vi "myDAQ Progression.vi"() -> ()   [LabVIEW 2010]
doc: "NI-K12 Lab style progress page with 5 parts."
uses:
  ActivityGuideEvents.ctl
  Utilities/myDAQ_State.ctl
  Utilities/AG Tab Action.ctl
  Utilities/myDAQmx/myDAQmx Create Channel/Create myDAQ AI.vi
  Utilities/myDAQmx/myDAQmx Read/myDAQmx Read Analog Value.vi
panel:
  in  "Reconnect to myDAQ":bool
  out "Connected":bool
  out "Searching for myDAQ":bool
  in  "Progress Bar":T1(radio)=enum."Apply 4"
  in  "Focus":bool
  in  "stop":bool
  in  "Leave":bool
  in  "Resources":path[](array[path])
  in  "TabButtonsRef":refnum<vi>
  out "DAQ error Info":string
  out "Error Count":u32
  out "Error Out":errorcluster
  out "Current State":T2=enum."Disconnect"
  out "DAQ Loop":i32=548
  in  "ActivityGuideEvents":T3
  in  "Tab Control":T4(tab)=enum."Part 3"
  out "Value 0":dbl
  out "Part 5":dbl
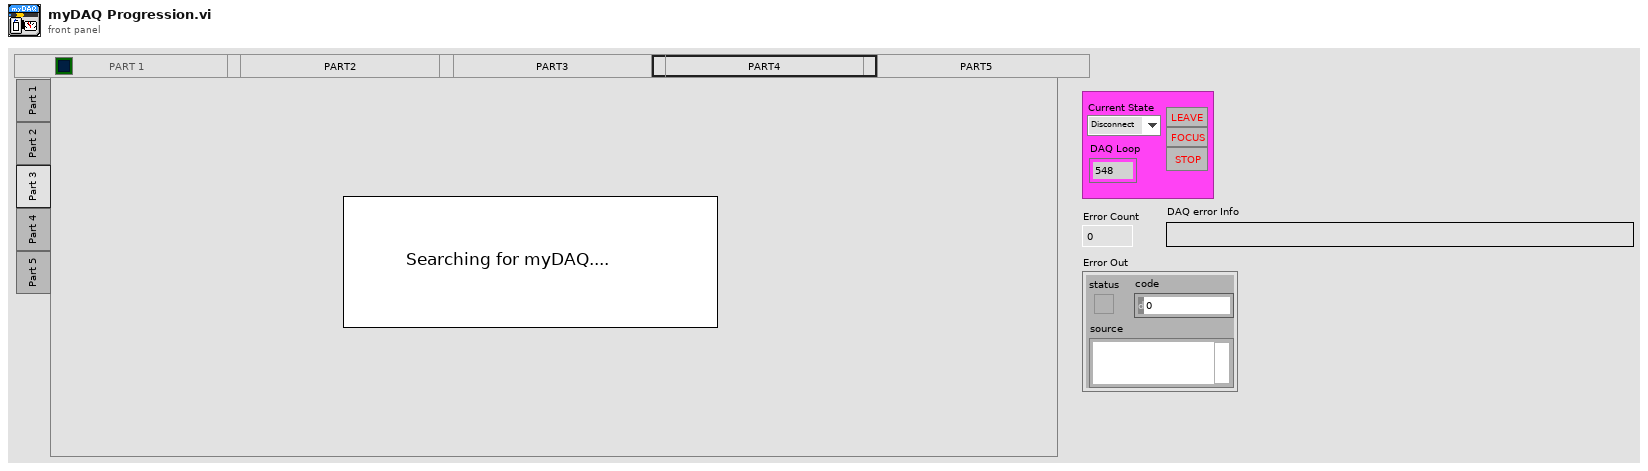
[diagram p1: front panel]
types:
  T1 = enum32{"Apply", "Apply 2", "Apply 3", "Apply 4", "Apply 5"}
  T2 = typedef "myDAQ_State.ctl" = enum16{"Initilize", "Connect", "Calibrate", "Communicate", "Wait", "Disconnect", "Error", "Close"}
  T3 = typedef "ActivityGuideEvents.ctl" = refnum<event-registration>
  T4 = enum32{"Part 1", "Part 2", "Part 3", "Part 4", "Part 5"}
  T5 = typedef "AG Tab Action.ctl" = enum16{"Initilize", "Select", "Blink", "Disable", "KeyFocus", "Set Description", "Hide", "NULL"}
  T6 = typedef "eventvkey.ctl" = enum16{"ASCII", "Enter", "Return", "Shift", "Ctrl", "Alt", "Cmd", "Opt", "Caps", "NumLock", "Clear", "Break", "Up", "Down", "Left", "Right", "Insert", "Delete", "Home", "End", "PageUp", "PageDown", "Escape", "Help", "Pause", "ScrollLock", "F1", "F2", "F3", "F4", "F5", "F6", "F7", "F8", "F9", "F10", "F11", "F12", "F13", "F14", "F15", "F16", "F17", "F18", "F19", "F20", "F21", "F22", "F23", "F24", "Play", "VolumeUp", "VolumeDown", "Mute", "Two Byte Char"}
  T7 = cluster{"Shift":bool, "Ctrl":bool, "Alt":bool, "Cmd":bool, "Opt":bool}
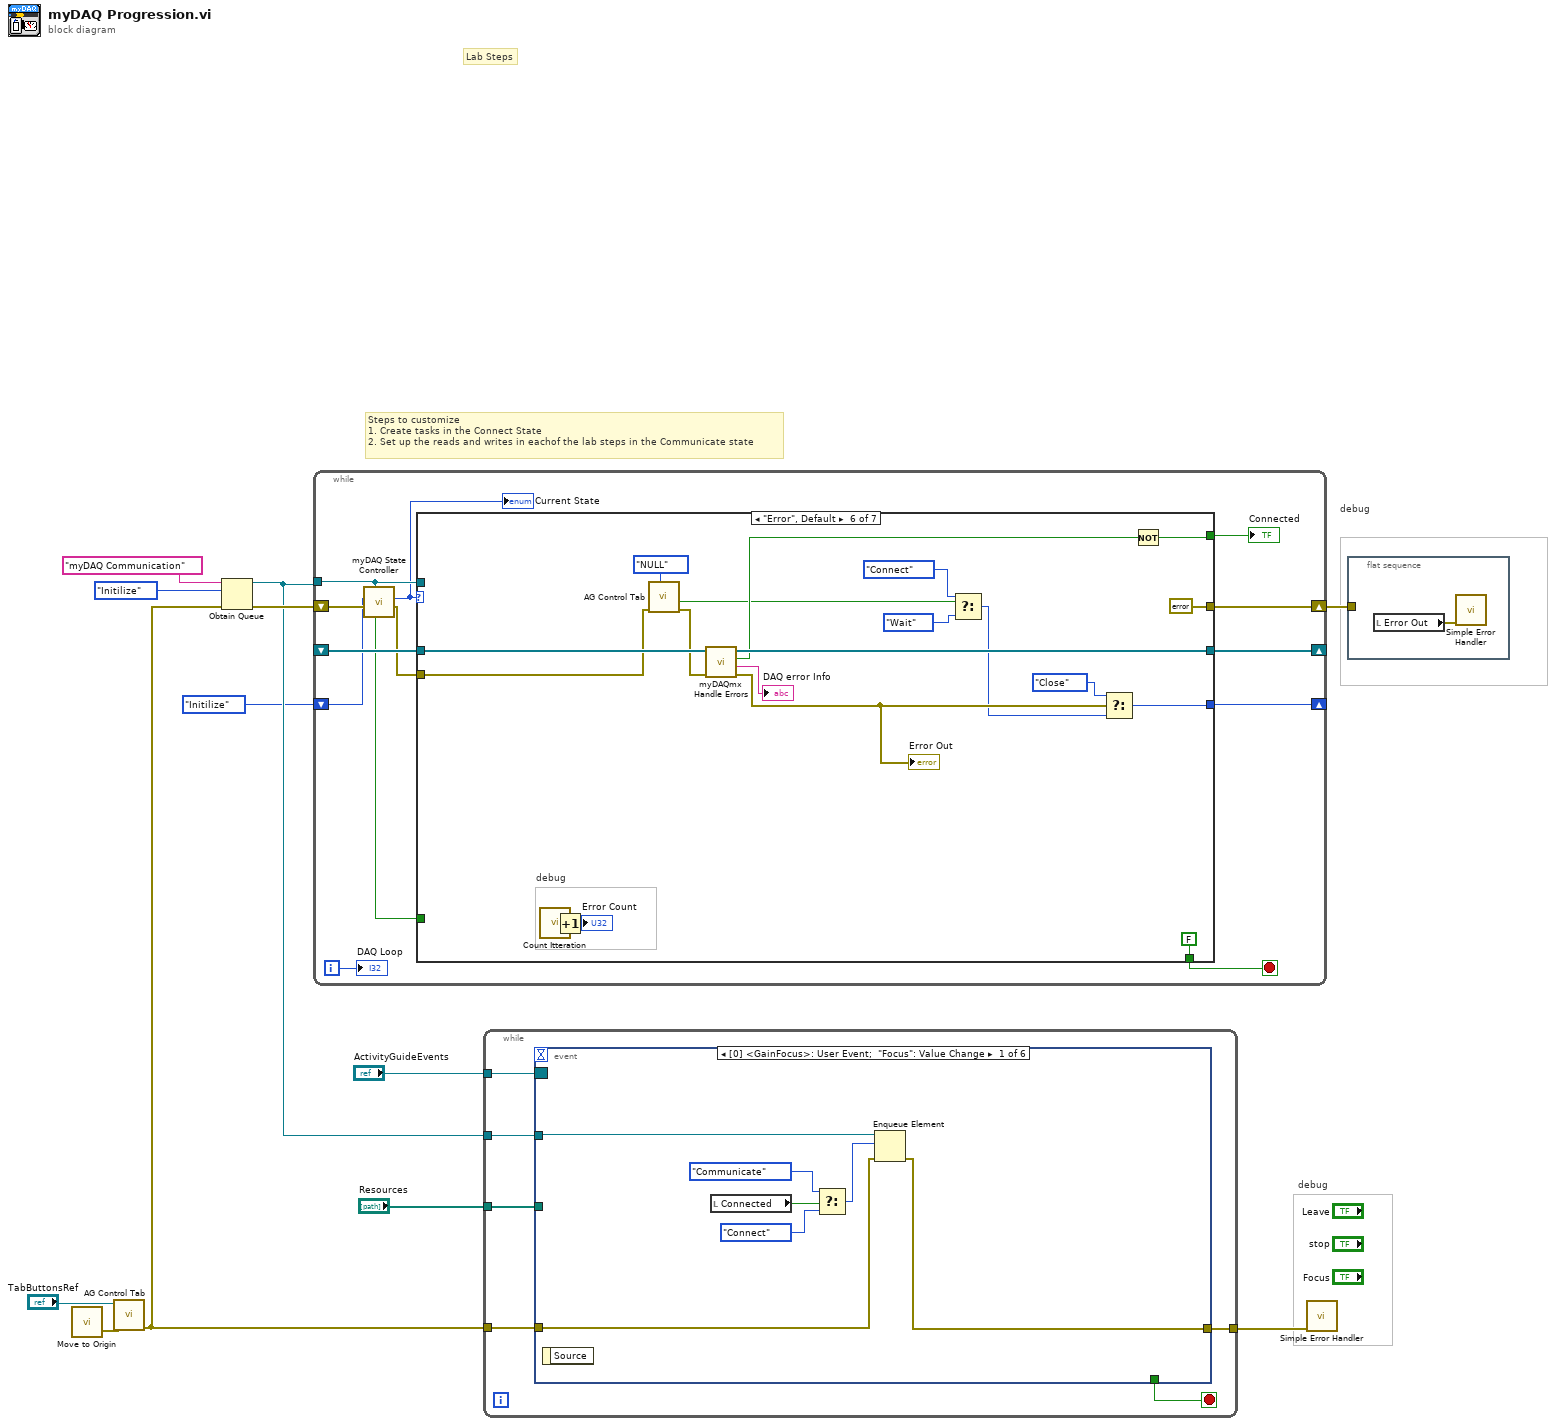
[diagram p0: block diagram]
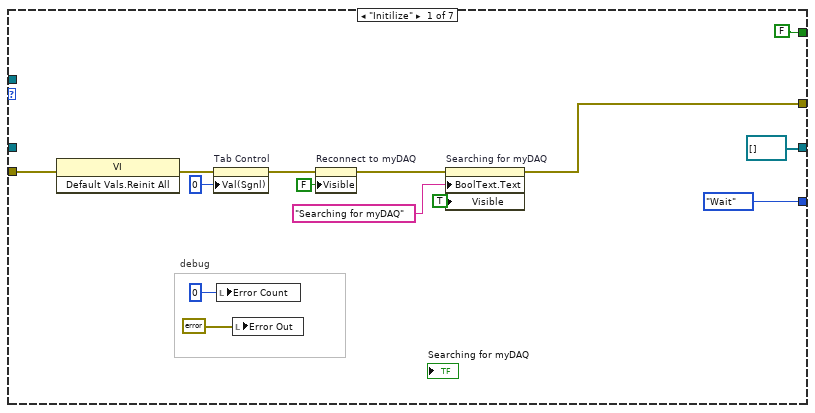
[diagram p2: hidden frame]
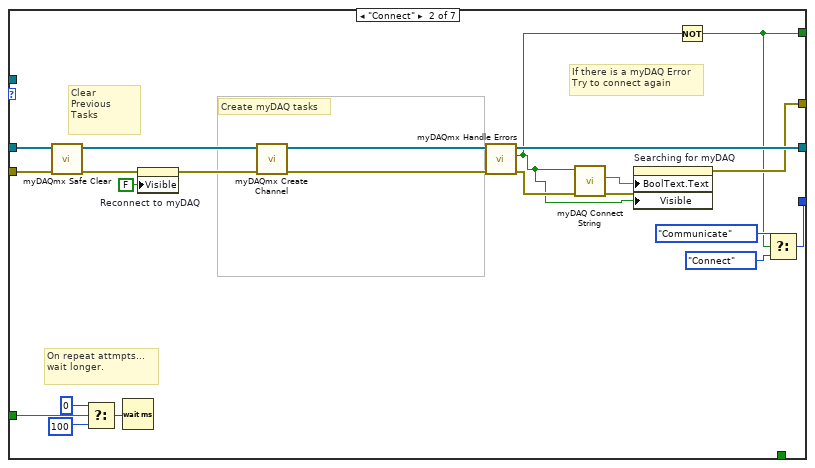
[diagram p3: hidden frame]
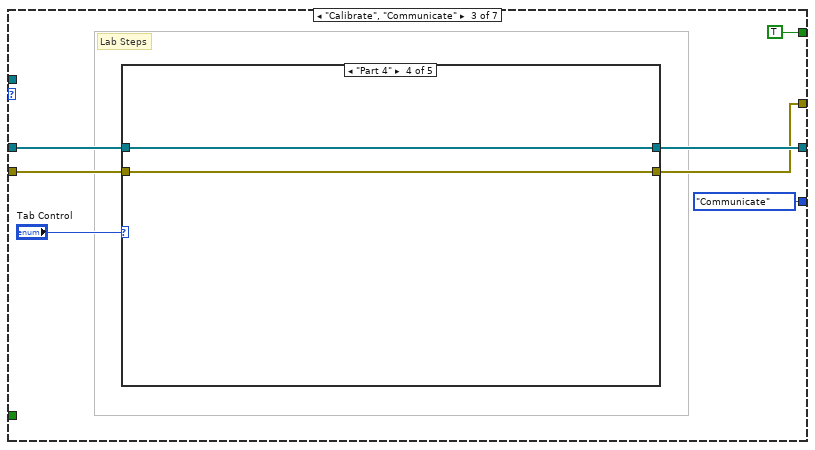
[diagram p4: hidden frame]
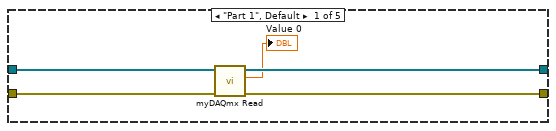
[diagram p5: hidden frame]
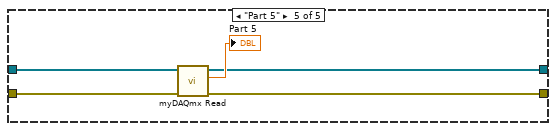
[diagram p8: hidden frame]
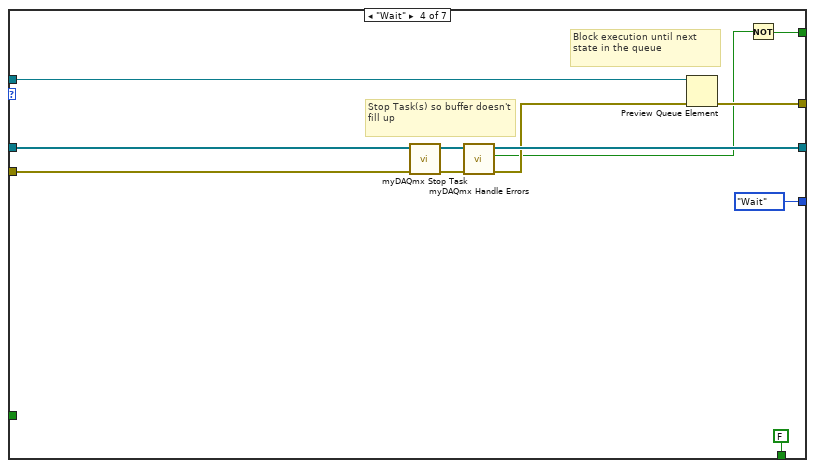
[diagram p9: hidden frame]
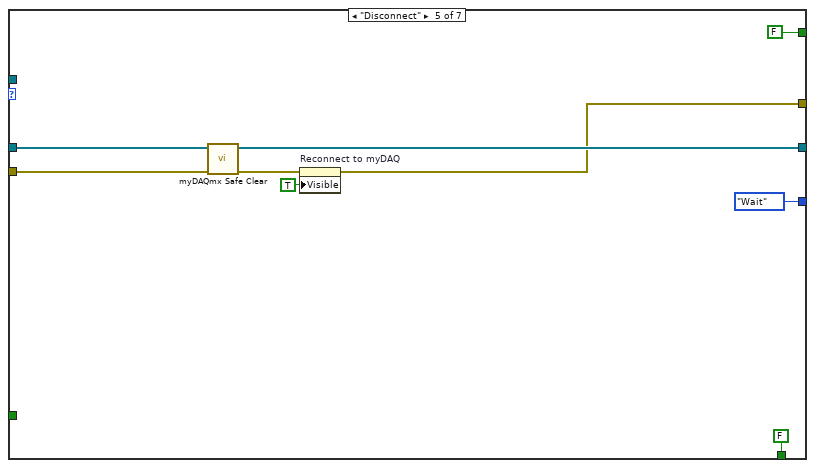
[diagram p10: hidden frame]
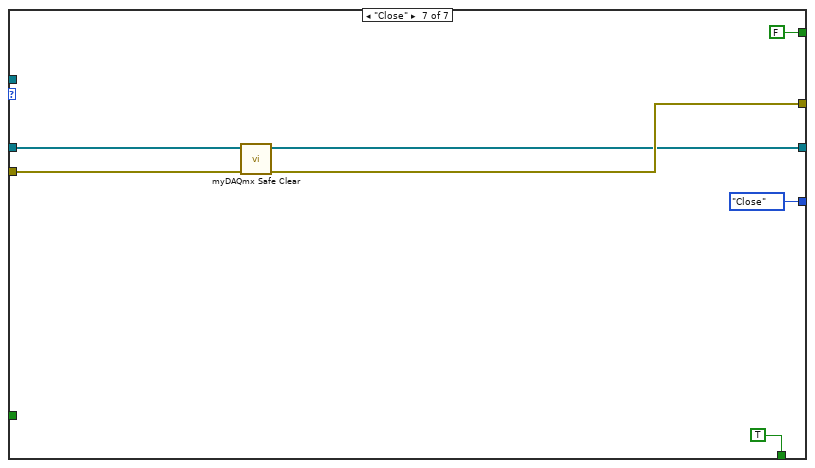
[diagram p11: hidden frame]
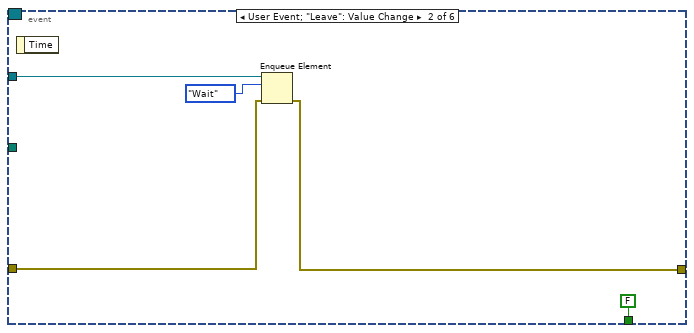
[diagram p12: hidden frame]
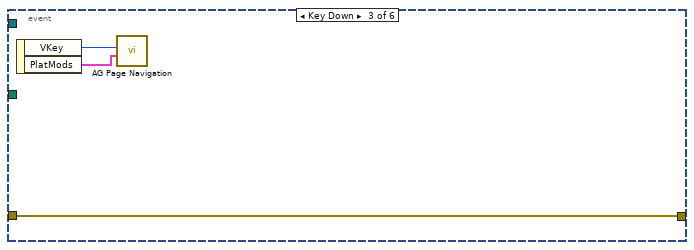
[diagram p13: hidden frame]
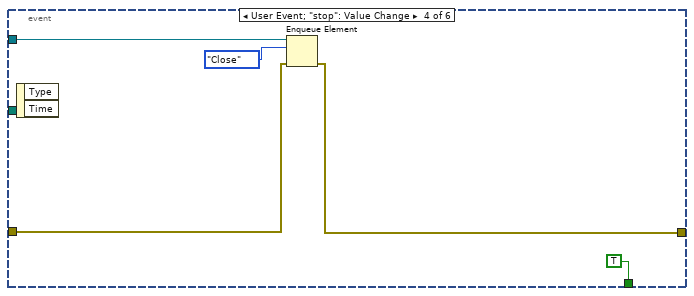
[diagram p14: hidden frame]
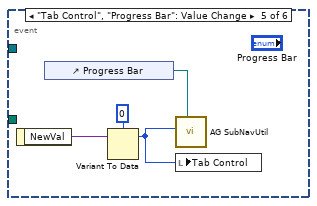
[diagram p15: hidden frame]
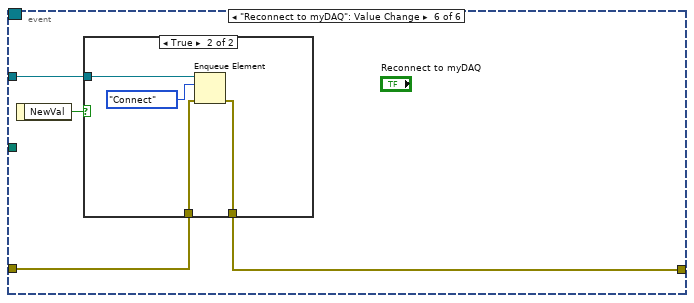
[diagram p16: hidden frame]
diagram:
  # "Steps to customize\n1. Create tasks in the Connect State\n2. Set up the reads and writes in eachof the lab steps in the Communicate state"
  # "Lab Steps"
  # "debug"
  # "debug"
  n1 = call "Move to Origin.vi"() -> ("Error Out"=w3:errorcluster)  [unwired: 3 in]
  n2 = call "AG Control Tab.vi"("error in (no error)"=w3, "TabButtonsRef"="TabButtonsRef") -> ("error out"=w2:errorcluster)  [unwired: 6 in, 3 out]
  n3 = Obtain Queue(name (unnamed)="myDAQ Communication", element data type=myDAQ_State."Initilize" ("Enum"), error in (no error)=w2) -> (queue out=w8:refnum<queue>, error out=w9:errorcluster)  [unwired: 2 in, 1 out]
  n4 = while {
    shift-right: [w24] -> _
    shift-left: myDAQ_State."Initilize" ("Enum") -> [w15]
    shift-right: [w23] -> _
    shift-left: _ -> [w20]
    shift-right: [w22] -> w6
    shift-left: w9 -> [w18]
    tunnel: w8 -> [w19]
    i -> [w21]
    stop <- w25 stop-if-true
    n5 = call "myDAQ State Controller.vi"("queue Ref"=w19, "error in (no error)"=w18, "Default State"=w15) -> ("error out"=w17:errorcluster, "State Out"=w16:T2, "New State?"=w14:bool)  [unwired: 6 in]
    "Current State" <- w16
    n6 = case shown="\"Error\", Default" w16 {
      tunnel: [_ _ _ FALSE FALSE FALSE TRUE] -> w25
      tunnel: [myDAQ_State."Wait" ("Enum") w61 myDAQ_State."Communicate" ("Enum") myDAQ_State."Wait" ("Enum") myDAQ_State."Wait" ("Enum") w113 myDAQ_State."Close" ("Enum")] -> w24
      tunnel: [refnum<k21>[] [] ("Task Array Out") w54 w66 w93 w102 w117 w126] -> w23
      tunnel: w20 -> [_ w56 w65 w85 w104 w118 w129]
      tunnel: [w29 w49 w62 w94 w97 errorcluster {"status"=FALSE, "code"=0, "source"=""} ("Error Out") w127] -> w22
      tunnel: w17 -> [w34 w55 w64 w88 w103 w110 w128]
      tunnel: w19 -> [_ _ _ w95 _ _ _]
      tunnel: w14 -> [_ w53 _ _ _ _ _]
      tunnel: [FALSE w43 TRUE w86 FALSE w109 FALSE] -> w13
      frame "Initilize" {
        # "debug"
        n7 = invoke class="VI" method="Default Vals.Reinit All"(error in=w34) -> (error out=w33:errorcluster)  [unwired: 2 in, 2 out]
        n8 = property on="Tab Control" class="TabCtl (strict)"(error in=w33, "Val(Sgnl)"=0 ("Error Count")) -> (error out=w30:errorcluster)  [unwired: 1 in, 1 out]
        n9 = local write "Error Count"(0 ("Error Count")) -> ()
        n10 = local write "Error Out"(errorcluster {"status"=FALSE, "code"=0, "source"=""} ("error in (no error)")) -> ()
        n11 = property on="Reconnect to myDAQ" class="Bool"(error in=w30, "Visible"=FALSE ("Visible (T)")) -> (error out=w31:errorcluster)  [unwired: 1 in, 1 out]
        n12 = property on="Searching for myDAQ" class="Bool"(error in=w31, "BoolText.Text"="Searching for myDAQ" ("Label.Text"), "Visible"=TRUE ("Visible (T)")) -> (error out=w29:errorcluster)  [unwired: 1 in, 1 out]
      }
      frame "Connect" {
        # "Create myDAQ tasks"
        # "If there is a myDAQ Error\nTry to connect again"
        # "On repeat attmpts... wait longer."
        # "Clear Previous Tasks"
        n13 = call "myDAQmx Safe Clear.vi"("error in (no error)"=w55, "task array in"=w56) -> ("error out"=w41:errorcluster, "task array out"=w40:refnum<k21>[])  [unwired: 8 in]
        n14 = Select(t=u32 0 ("milliseconds to wait"), s=w53, f=u32 100 ("milliseconds to wait")) -> (s? t:f=w59:u32)
        n15 = Wait (ms)(milliseconds to wait=w59) -> ()  [unwired: 1 out]
        n16 = property on="Reconnect to myDAQ" class="Bool"(error in=w41, "Visible"=FALSE ("Visible (T)")) -> (error out=w44:errorcluster)  [unwired: 1 in, 1 out]
        n17 = call-poly "myDAQmx Create Channel.vi"("error in (no error)"=w44, "task array in (none)"=w40) -> ("error out"=w46:errorcluster, "task array out"=w47:refnum<k21>[])  [unwired: 8 in]
        n18 = call "myDAQmx Handle Errors.vi"("Error In"=w46, "Task Array In"=w47) -> ("Error Out"=w52:errorcluster, "Require Reconnect?"=w42:bool, "Task Array Out"=w54:refnum<k21>[])  [unwired: 6 in, 1 out]
        n19 = call "myDAQ Connect String.vi"("error in (no error)"=w52, "Searching? (T)"=w42) -> ("error out"=w51:errorcluster, "myDAQ String"=w50:string)  [unwired: 8 in]
        n20 = property on="Searching for myDAQ" class="Bool"(error in=w51, "BoolText.Text"=w50, "Visible"=w42) -> (error out=w49:errorcluster)  [unwired: 1 in, 1 out]
        n21 = Not(x=w42) -> (.not. x?=w43:bool)
        n22 = Select(t=myDAQ_State."Communicate" ("Enum"), s=w43, f=myDAQ_State."Connect" ("Enum")) -> (s? t:f=w61:T2)
      }
      frame "Calibrate", "Communicate" {
        # "Lab Steps"
        n23 = case shown="\"Part 4\"" "Tab Control" {
          tunnel: [w70 w74 w76 w78 w81] -> w62
          tunnel: [w71 w75 w77 w79 w80] -> w66
          tunnel: w65 -> [w73 w75 w77 w79 w83]
          tunnel: w64 -> [w72 w74 w76 w78 w82]
          frame "Part 1", Default {
            n24 = call-poly "myDAQmx Read.vi"("error in (no error)"=w72, "task array in"=w73) -> ("error out"=w70:errorcluster, "value 0"=→"Value 0":dbl, "task array out"=w71:refnum<k21>[])  [unwired: 6 in, 1 out]
          }
          frame "Part 2" {
          }
          frame "Part 3" {
          }
          frame "Part 4" {
          }
          frame "Part 5" {
            n25 = call-poly "myDAQmx Read.vi"("error in (no error)"=w82, "task array in"=w83) -> ("error out"=w81:errorcluster, "value 0"=→"Part 5":dbl, "task array out"=w80:refnum<k21>[])  [unwired: 6 in, 1 out]
          }
        }
      }
      frame "Wait" {
        # "Block execution until next state in the queue"
        # "Stop Task(s) so buffer doesn't fill up"
        n26 = call "myDAQmx Stop Task.vi"("error In"=w88, "task array in"=w85) -> ("Error Out"=w89:errorcluster, "task array out"=w90:refnum<k21>[])  [unwired: 8 in]
        n27 = call "myDAQmx Handle Errors.vi"("Error In"=w89, "Task Array In"=w90) -> ("Error Out"=w92:errorcluster, "Require Reconnect?"=w87:bool, "Task Array Out"=w93:refnum<k21>[])  [unwired: 6 in, 1 out]
        n28 = Preview Queue Element(queue=w95, error in (no error)=w92) -> (error out=w94:errorcluster)  [unwired: 1 in, 3 out]
        n29 = Not(x=w87) -> (.not. x?=w86:bool)
      }
      frame "Disconnect" {
        n30 = call "myDAQmx Safe Clear.vi"("error in (no error)"=w103, "task array in"=w104) -> ("error out"=w98:errorcluster, "task array out"=w102:refnum<k21>[])  [unwired: 8 in]
        n31 = property on="Reconnect to myDAQ" class="Bool"(error in=w98, "Visible"=TRUE ("Visible (T)")) -> (error out=w97:errorcluster)  [unwired: 1 in, 1 out]
      }
      frame "Error", Default {
        # "debug"
        n32 = call "Count Itteration.vi"() -> ("Itteration"=w123:i32)  [unwired: 7 in, 1 out]
        n33 = Increment(x=w123) -> (x+1=→"Error Count":i32)
        n34 = call "AG Control Tab.vi"("Action (Init)"=AG_Tab_Action."NULL", "error in (no error)"=w110) -> ("error out"=w111:errorcluster, "Selected?"=w112:bool)  [unwired: 6 in, 2 out]
        n35 = call "myDAQmx Handle Errors.vi"("Error In"=w111, "Task Array In"=w118) -> ("Error Out"=w115:errorcluster, "DAQ error Info"=→"DAQ error Info":string, "Require Reconnect?"=w116:bool, "Task Array Out"=w117:refnum<k21>[])  [unwired: 6 in]
        "Error Out" <- w115
        n36 = Select(t=myDAQ_State."Connect", s=w112, f=myDAQ_State."Wait" ("t")) -> (s? t:f=w107:T2)
        n37 = Select(t=myDAQ_State."Close", s=w115, f=w107) -> (s? t:f=w113:T2)
        n38 = Not(x=w116) -> (.not. x?=w109:bool)
      }
      frame "Close" {
        n39 = call "myDAQmx Safe Clear.vi"("error in (no error)"=w128, "task array in"=w129) -> ("error out"=w127:errorcluster, "task array out"=w126:refnum<k21>[])  [unwired: 8 in]
      }
    }
    "Connected" <- w13
    "DAQ Loop" <- w21
  }
  n40 = while {
    tunnel: "ActivityGuideEvents" -> [w137]
    tunnel: w8 -> [w135]
    tunnel: "Resources" -> [w134]
    tunnel: w2 -> [w133]
    tunnel: [w132] -> w1
    stop <- w136 stop-if-true
    n41 = event shown="[0] <GainFocus>: User Event;  \"Focus\": Value Change" {
      selector: w137 -> [_ _ _ _ _ _]
      dyn-events: _ -> [_ _ _ _ _ _]
      timeout: _ -> [_ _ _ _ _ _]
      tunnel: [_ FALSE _ TRUE _ _] -> w136
      tunnel: w135 -> [w144 w149 _ w156 _ w165]
      tunnel: w134 -> [_ _ _ _ _ _]
      tunnel: w133 -> [w141 w146 w151 w154 _ w164]
      tunnel: [w140 w145 w151 w153 _ w163] -> w132
      event User Event; "Focus": Value Change {
        n42 = event-data() -> ()  [unwired: 1 in, 1 out]
        n43 = local read "Connected"() -> (w139:bool)
        n44 = Select(t=myDAQ_State."Communicate" ("Enum"), s=w139, f=myDAQ_State."Connect" ("Enum")) -> (s? t:f=w142:T2)
        n45 = Enqueue Element(queue=w144, element=w142, error in (no error)=w141) -> (error out=w140:errorcluster)  [unwired: 1 in, 2 out]
      }
      event User Event; "Leave": Value Change {
        n46 = event-data() -> ()  [unwired: 1 in, 1 out]
        n47 = Enqueue Element(queue=w149, element=myDAQ_State."Wait", error in (no error)=w146) -> (error out=w145:errorcluster)  [unwired: 1 in, 2 out]
      }
      event Key Down {
        n48 = event-data() -> ("VKey"=w152:T6, "PlatMods"=w150:T7)  [unwired: 1 in]
        n49 = call "AG Page Navigation.vi"("PlatMods"=w150, "VKey"=w152) -> ()  [unwired: 8 in, 2 out]
      }
      event User Event; "stop": Value Change {
        n50 = event-data() -> ()  [unwired: 1 in, 2 out]
        n51 = Enqueue Element(queue=w156, element=myDAQ_State."Close", error in (no error)=w154) -> (error out=w153:errorcluster)  [unwired: 1 in, 2 out]
      }
      event "Tab Control", "Progress Bar": Value Change {
        n52 = event-data() -> ("NewVal"=w160:variant)  [unwired: 1 in]
        n53 = control-ref of="Progress Bar"() -> (w161:refnum<vi>)
        n54 = Variant To Data(Variant=w160, type=0) -> (data=w158:i32)  [unwired: 1 in, 1 out]
        n55 = call "AG SubNavUtil.vi"("Progress Ref"=w161, "NewVal"=w158) -> ()  [unwired: 9 in, 1 out]
        n56 = local write "Tab Control"(w158) -> ()
      }
      event "Reconnect to myDAQ": Value Change {
        n57 = event-data() -> ("NewVal"=w162:bool)  [unwired: 1 in]
        n58 = case shown="True" w162 {
          tunnel: w165 -> [_ w170]
          tunnel: w164 -> [w166 w168]
          tunnel: [w166 w167] -> w163
          frame False {
          }
          frame True {
            n59 = Enqueue Element(queue=w170, element=myDAQ_State."Connect", error in (no error)=w168) -> (error out=w167:errorcluster)  [unwired: 1 in, 2 out]
          }
        }
      }
    }
  }
  n60 = call <vilib>:"Simple Error Handler.vi"("error in (no error)"=w1) -> ()  [unwired: 4 in, 5 out]
  n61 = flat-sequence {
    tunnel: w6 -> [_]
    frame #0 {
      n62 = local read "Error Out"() -> (w171:errorcluster)
      n63 = call <vilib>:"Simple Error Handler.vi"("error in (no error)"=w171) -> ()  [unwired: 4 in, 5 out]
    }
  }
